vi "Send_A_Status.vi"(8 "error in (no error)":errorcluster, 10 "Status":string, 11 "A_Actor in":refnum<class "A_Actor.lvclass">) -> (0 "error out":errorcluster, 3 "A_Actor out":refnum<class "A_Actor.lvclass">)   [LabVIEW 2025, in "A_Actor.lvlib" / "A_Actor.lvclass"]
uses:
  A_Actor.lvclass
  <vilib>/ActorFramework/Actor/Actor.lvclass/Actor.ctl
  <vilib>/ActorFramework/Message Enqueuer/Message Enqueuer.lvclass/Message Enqueuer.ctl
  A_Actor.lvclass/A_Actor.ctl
  A_Actor Messages/A_msg Msg/A_msg Msg.lvclass/A_msg Msg.ctl
  <vilib>/ActorFramework/Message Enqueuer/Init from Existing Queue.vi
  <vilib>/ActorFramework/Message Enqueuer/Enqueue.vi
  A_Actor Messages/A_msg Msg/A_msg Msg.lvclass
  <vilib>/ActorFramework/Message Priority Queue/Priority Enqueue.vi
  <vilib>/ActorFramework/Message Enqueuer/Message Enqueuer.lvclass
  C:/Program Files (x86)/National Instruments/LabVIEW 2025/vi.lib/ActorFramework/Actor/Actor.lvclass
  C:/Users/halstead_rideriver/Documents/Labview_Practice/Tasks_Actor/A_Actor/A_Actor.lvclass
  <vilib>/ActorFramework/Actor/Actor.lvclass
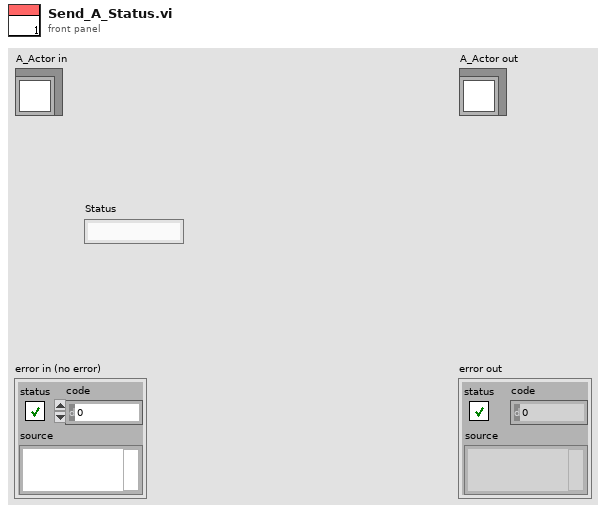
[diagram p1: front panel]
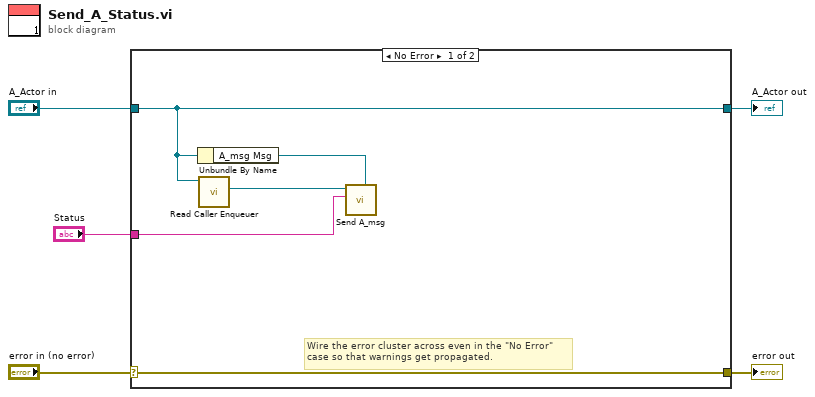
[diagram p0: block diagram]
diagram:
  n1 = case shown="No Error" "error in (no error)" {
    selector: "error in (no error)" -> [w10 w12]
    tunnel: [w10 w12] -> w4
    tunnel: [w9 w11] -> w2
    tunnel: "A_Actor in" -> [w9 w11]
    tunnel: "Status" -> [w6 _]
    frame No Error {
      # "Wire the error cluster across even in the \"No Error\"\ncase so that warnings get propagated."
      n2 = Unbundle By Name(w9) -> ("A_msg Msg"=w8:refnum<class "A_msg Msg.lvclass">)
      n3 = call <vilib>:"Read Caller Enqueuer.vi"("Actor"=w9) -> ("Caller Enqueuer"=w7:refnum<class "Message Enqueuer.lvclass">)  [unwired: 10 in]
      n4 = call "Send A_msg.vi"("Message Type"=w8, "Status"=w6, "Message Enqueuer"=w7) -> ()  [unwired: 7 in, 2 out]
    }
    frame Error {
    }
  }
  "error out" <- w4
  "A_Actor out" <- w2
